vi "250224_Nikon_CheckStatus.vi"(8 "error in":errorcluster caption="entrée d'erreur", 11 "NikonTi2AxLib.INikonTi2AxMicroscope":refnum<k7>) -> (0 "error out":errorcluster={"status"=TRUE, "code"=-9, "source"="Exception occured in Nikon.Ti2.Microscope.1: Failed in 231026_NikonTi2_Indicators_v2.vi"} caption="sortie d'erreur", 2 "Nikon Cluster":T1, 3 "reference out":refnum<k7>)   [LabVIEW 2025]
doc: "This vi checks the current status of the microscope. One can add some extra devices such as fluorescence cube turret.\nThe automation should be open and close outside of this vi"
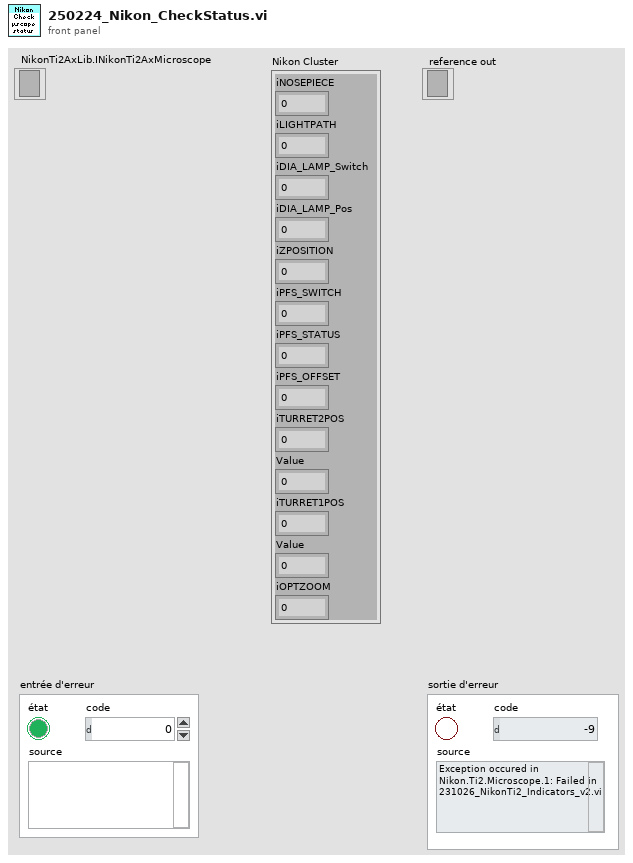
[diagram p1: front panel]
types:
  T1 = cluster{"iNOSEPIECE":i32, "iLIGHTPATH":i32, "iDIA_LAMP_Switch":i32, "iDIA_LAMP_Pos":i32, "iZPOSITION":i32, "iPFS_SWITCH":i32, "iPFS_STATUS":i32, "iPFS_OFFSET":i32, "iTURRET2POS":i32, "Value":i32, "iTURRET1POS":i32, "Value":i32, "iOPTZOOM":i32}
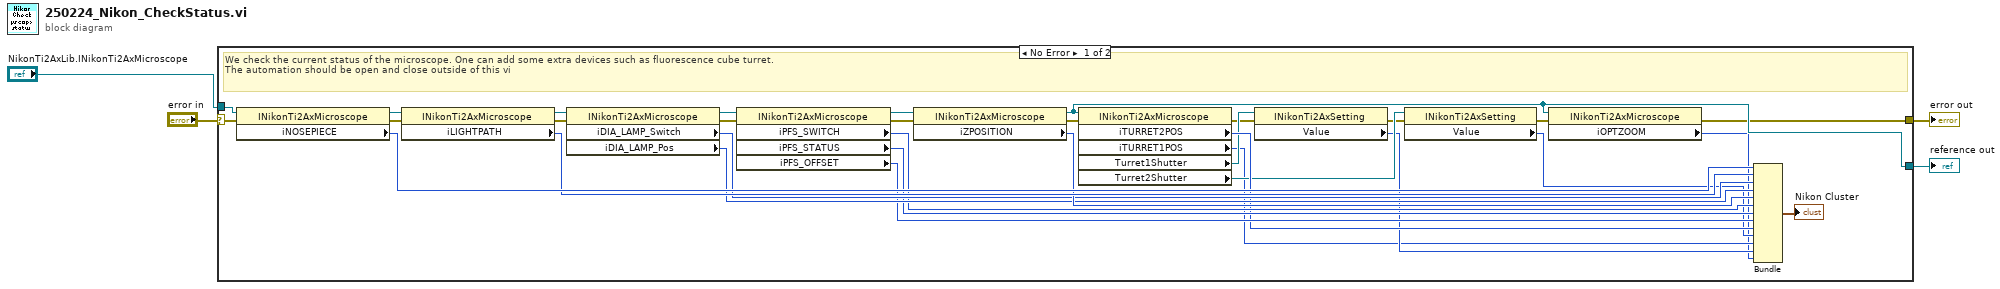
[diagram p0: block diagram]
diagram:
  n1 = case shown="No Error" "error in" {
    selector: "error in" -> [w19 w38]
    tunnel: [w7 w38] -> w3
    tunnel: "NikonTi2AxLib.INikonTi2AxMicroscope" -> [w20 w37]
    tunnel: [w9 w37] -> w2
    frame No Error {
      # "We check the current status of the microscope. One can add some extra devices such as fluorescence cube turret.\nThe automation should be open and close outside of this vi"
      n2 = property class="INikonTi2AxMicroscope"(reference=w20, error in=w19) -> (reference out=w33:refnum<k7>, error out=w32:errorcluster, "iNOSEPIECE"=w36:i32)
      n3 = property class="INikonTi2AxMicroscope"(reference=w33, error in=w32) -> (reference out=w31:refnum<k7>, error out=w30:errorcluster, "iLIGHTPATH"=w35:i32)
      n4 = property class="INikonTi2AxMicroscope"(reference=w31, error in=w30) -> (reference out=w27:refnum<k7>, error out=w26:errorcluster, "iDIA_LAMP_Switch"=w29:i32, "iDIA_LAMP_Pos"=w28:i32)
      n5 = property class="INikonTi2AxMicroscope"(reference=w27, error in=w26) -> (reference out=w24:refnum<k7>, error out=w25:errorcluster, "iPFS_SWITCH"=w23:i32, "iPFS_STATUS"=w22:i32, "iPFS_OFFSET"=w21:i32)
      n6 = property class="INikonTi2AxMicroscope"(reference=w24, error in=w25) -> (reference out=w9:refnum<k7>, error out=w17:errorcluster, "iZPOSITION"=w34:i32)
      n7 = property class="INikonTi2AxMicroscope"(reference=w9, error in=w17) -> (error out=w11:errorcluster, "iTURRET2POS"=w18:i32, "iTURRET1POS"=w12:i32, "Turret1Shutter"=w16:refnum<k7>, "Turret2Shutter"=w15:refnum<k7>)  [unwired: 1 out]
      n8 = property class="INikonTi2AxSetting"(reference=w16, error in=w11) -> (error out=w10:errorcluster, "Value"=w13:i32)  [unwired: 1 out]
      n9 = property class="INikonTi2AxSetting"(reference=w15, error in=w10) -> (error out=w8:errorcluster, "Value"=w14:i32)  [unwired: 1 out]
      n10 = property class="INikonTi2AxMicroscope"(reference=w9, error in=w8) -> (error out=w7:errorcluster, "iOPTZOOM"=w6:i32)  [unwired: 1 out]
      n11 = Bundle("iNOSEPIECE"=w36, "iLIGHTPATH"=w35, "iDIA_LAMP_Switch"=w29, "iDIA_LAMP_Pos"=w28, "iZPOSITION"=w34, "iPFS_SWITCH"=w23, "iPFS_STATUS"=w22, "iPFS_OFFSET"=w21, "iTURRET2POS"=w18, "Value"=w14, "iTURRET1POS"=w12, "Value"=w13, "iOPTZOOM"=w6) -> (→"Nikon Cluster":T1)  [unwired: 1 in]
    }
    frame Error {
    }
  }
  "error out" <- w3
  "reference out" <- w2
